vi "Edge Detection.vi"(5 "reset? (True)":bool=TRUE, 6 "sampling frequency [Hz]":dbl=11025.0, 7 "missing pulses? (no:F)":bool, 8 "slope (Rise)":enum16{"Rise", "Fall"}(ring), 9 "pulse width (2)":i32=2, 10 "threshold (0.0)":dbl format="%.2f", 11 "x[n]":dbl[](array[numeric]) format="%.2f") -> (1 "number of pulses":i32, 3 "pulse positions [s]":dbl[](array[numeric]) format="%.2f")   [LabVIEW 2017, in "SoundVib_TachProcess.lvlib"]
doc: "Detects the edges in the tachometer pulses contained in <B>x[n]</B> that cross <B>threshold</B>. Perform edge detection to determine the tachometer pulse position. The VI recognizes the points where the signal crosses <B>threshold</B> and <B>x[n]</B> as edges. The VI returns the locations of the detected edges in <B>pulse positions [s]</B>."
uses:
  <vilib>/addons/Sound and Vibration/Order Analysis/Tach Process/SoundVib_TachProcess.lvlib
  <vilib>/Analysis/8numeric.llb/Threshold Detector.vi
panel:
  # "Edge Detection"
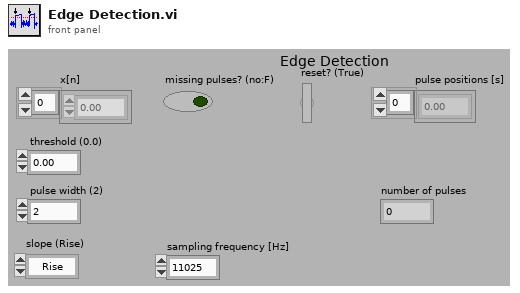
[diagram p1: front panel]
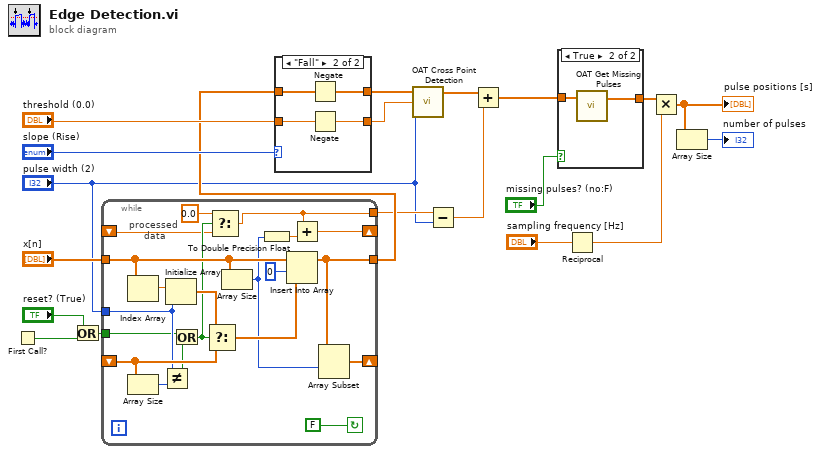
[diagram p0: block diagram]
diagram:
  n1 = First Call?() -> (First Call?: T/F=w1:bool)
  n2 = Or(x="reset? (True)", y=w1) -> (x .or. y?=w9:bool)
  n3 = while {
    shift-right: [w33] -> _
    shift-left: _ -> [w38]
    tunnel: "x[n]" -> [w32]
    tunnel: "pulse width (2)" -> [w36]
    tunnel: [w29] -> w10
    tunnel: w9 -> [w34]
    shift-right: [w28] -> _
    shift-left: _ -> [w25]
    tunnel: [w23] -> w6
    stop <- FALSE continue-if-true
    # "processed\n     data"
    n4 = Index Array(array=w32) -> (element=w39:dbl)  [unwired: 1 in]
    n5 = Array Size(array=w38) -> (size(s)=w37:i32)
    n6 = Not Equal?(x=w36, y=w37) -> (x != y?=w35:bool)
    n7 = Initialize Array(w39, w36) -> (w27:dbl[])
    n8 = Or(x=w34, y=w35) -> (x .or. y?=w26:bool)
    n9 = Select(t=w27, s=w26, f=w38) -> (s? t:f=w31:dbl[])
    n10 = Select(t=0.0, s=w26, f=w25) -> (s? t:f=w23:dbl)
    n11 = Array Size(array=w32) -> (size(s)=w22:i32)
    n12 = To Double Precision Float(number=w22) -> (double precision float=w21:dbl)
    n13 = Insert Into Array(array=w32, index=0 ("Index"), new element=w31) -> (w29:dbl[])
    n14 = Add(x=w23, y=w21) -> (x+y=w28:dbl)
    n15 = Array Subset(array=w29, index=w22) -> (w33:dbl[])  [unwired: 1 in]
  }
  n16 = case shown="\"Fall\"" "slope (Rise)" {
    tunnel: "threshold (0.0)" -> [w41 w44]
    tunnel: w10 -> [w42 w46]
    tunnel: [w42 w45] -> w17
    tunnel: [w41 w43] -> w19
    frame "Rise", Default {
    }
    frame "Fall" {
      n17 = Negate(x=w46) -> (-x=w45:dbl[])
      n18 = Negate(x=w44) -> (-x=w43:dbl)
    }
  }
  n19 = call <vilib>:"OAT Cross Point Detection.vi"("pulse width (2)"="pulse width (2)", "threshold (0)"=w19, "data in"=w17) -> ("edge position"=w7:dbl[])  [unwired: 1 in]
  n20 = Subtract(x=w6, y="pulse width (2)") -> (x-y=w4:dbl)
  n21 = Add(x=w7, y=w4) -> (x+y=w8:dbl[])
  n22 = case shown="True" "missing pulses? (no:F)" {
    tunnel: w8 -> [w47 w49]
    tunnel: [w47 w48] -> w15
    frame False {
    }
    frame True {
      n23 = call <vilib>:"OAT Get Missing Pulses.vi"("pulse positions"=w49) -> ("modified pulse positions"=w48:dbl[])  [unwired: 1 in, 1 out]
    }
  }
  n24 = Reciprocal(x="sampling frequency [Hz]") -> (1/x=w3:dbl)
  n25 = Multiply(x=w15, y=w3) -> (x*y=w13:dbl[])
  "pulse positions [s]" <- w13
  n26 = Array Size(array=w13) -> (size(s)=→"number of pulses":i32)
